vi "Wait Raw.vi"(8 "error in (no error)":errorcluster, 11 "Event in":refnum<class "Event.lvclass">) -> (0 "error out":errorcluster, 3 "Event out":refnum<class "Event.lvclass">)   [LabVIEW 2010]
doc: "Get data received as a raw buffer."
uses:
  <vilib>/MDSplus/Classes/Event_Class/Event.lvclass
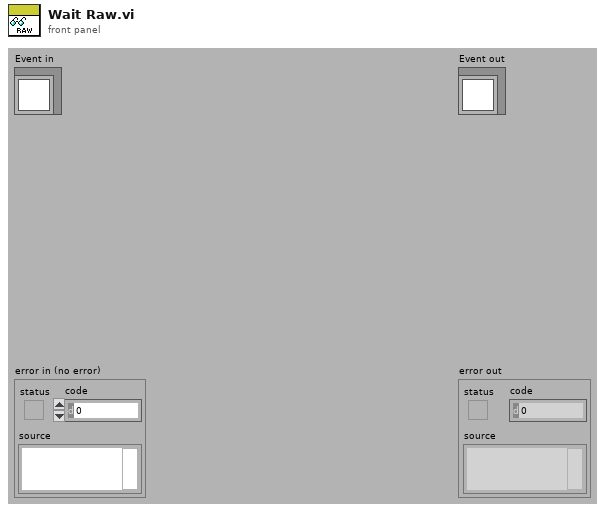
[diagram p1: front panel]
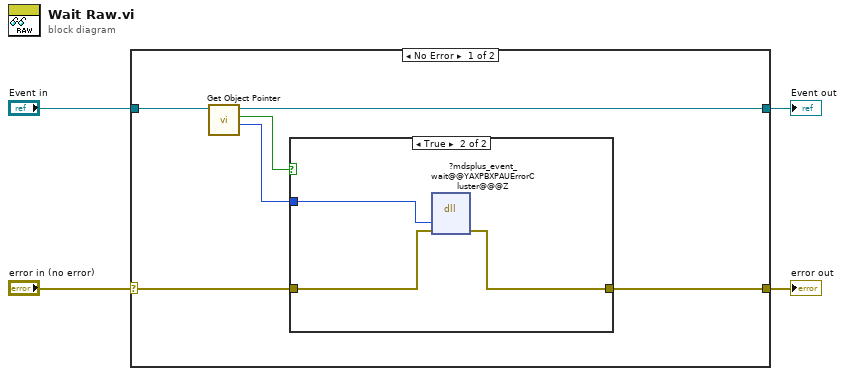
[diagram p0: block diagram]
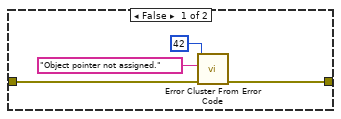
[diagram p2: hidden frame]
diagram:
  n1 = case shown="No Error" "error in (no error)" {
    selector: "error in (no error)" -> [w6 w19]
    tunnel: [w5 w19] -> w3
    tunnel: [w9 w18] -> w1
    tunnel: "Event in" -> [w10 w18]
    frame No Error {
      n2 = call-dynamic "Get Object Pointer.vi"("Event in"=w10) -> ("Object Pointer"=w7:i64, "Assigned object pointer?"=w8:bool, "Event out"=w9:refnum<class "Event.lvclass">)  [unwired: 8 in]
      n3 = case shown="True" w8 {
        tunnel: w7 -> [_ w17]
        tunnel: w6 -> [w12 w16]
        tunnel: [w11 w15] -> w5
        frame False {
          n4 = call <vilib>:"Error Cluster From Error Code.vi"("error in (no error)"=w12, "error message (\"\")"="Object pointer not assigned." ("error message (\"\")"), "error code (0)"=42) -> ("error out"=w11:errorcluster)  [unwired: 6 in]
        }
        frame True {
          n5 = dll-call lib="MDSobjectsLVShr" fn="?mdsplus_event_wait@@YAXPBXPAUErrorCluster@@@Z"("lvEventPtr"=w17, "error"=w16) -> ("error"=w15:errorcluster)  [unwired: 5 in, 2 out]
        }
      }
    }
    frame Error {
    }
  }
  "error out" <- w3
  "Event out" <- w1
